vi "JoinGame.vi"(8 "error in (no error)":errorcluster, 10 "PlayerName":string, 11 "CS++GoBangServer in":refnum<class "CS++GoBangServer.lvclass">) -> (0 "error out":errorcluster, 3 "CS++GoBangServer out":refnum<class "CS++GoBangServer.lvclass">)   [LabVIEW 2014, in "GoBang.lvlib" / "CS++GoBangServer.lvclass"]
uses:
  CS++GoBangServer.lvclass
  typdefs/GameState.ctl
  CS++GoBangServer.lvclass/CS++GoBangServer.ctl
  GoBang.lvlib
panel:
  in  "Color(True=White)":bool
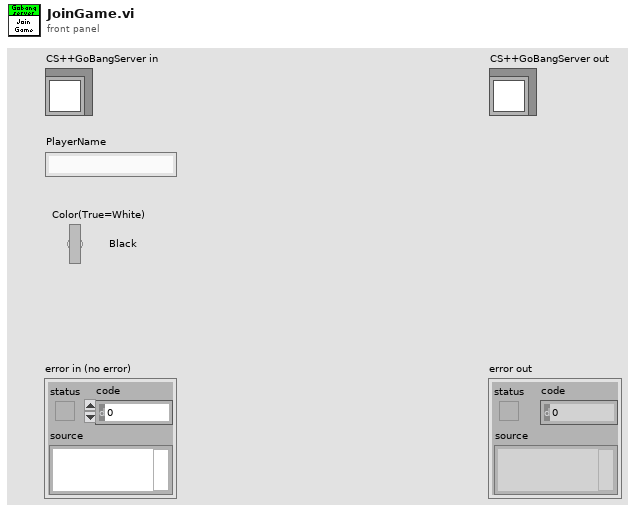
[diagram p1: front panel]
types:
  T1 = typedef "GoBang.lvlib/GameState.ctl" = enum16{"Waiting for opponent", "White to move", "Black to move", "Game over, white won", "Game over, black won"}
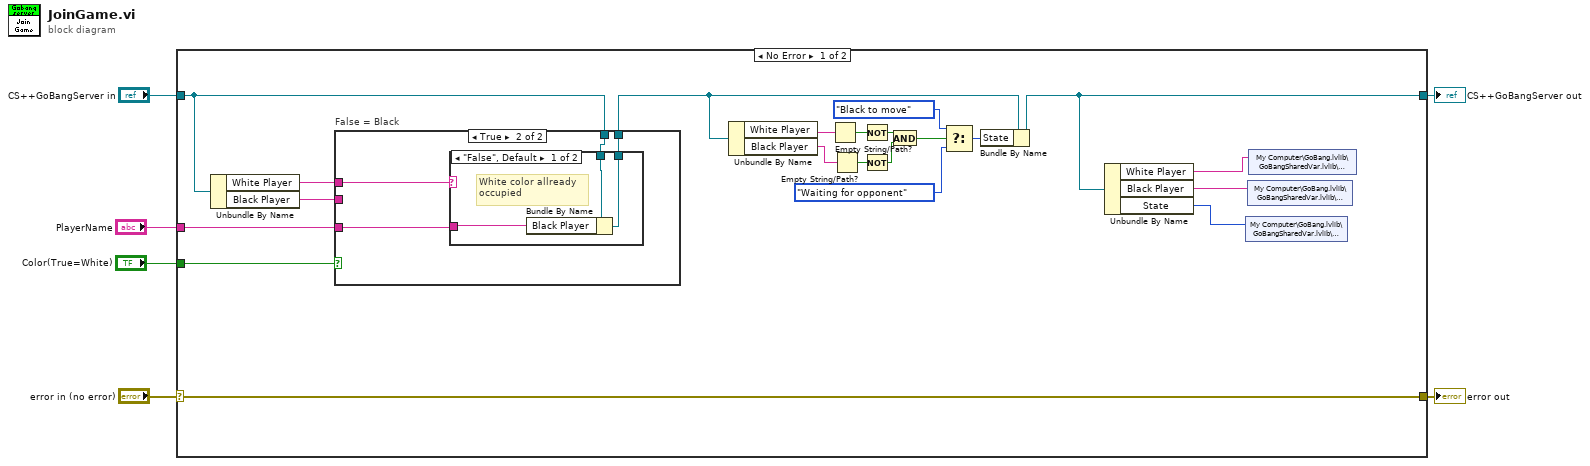
[diagram p0: block diagram]
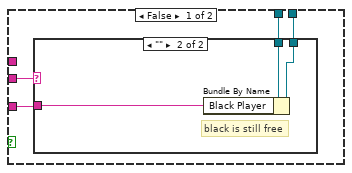
[diagram p2: hidden frame]
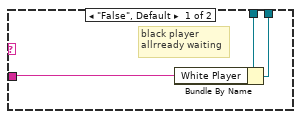
[diagram p3: hidden frame]
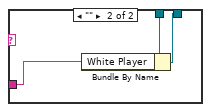
[diagram p4: hidden frame]
diagram:
  n1 = case shown="No Error" "error in (no error)" {
    selector: "error in (no error)" -> [w22 w49]
    tunnel: [w22 w49] -> w5
    tunnel: [w11 w48] -> w3
    tunnel: "CS++GoBangServer in" -> [w25 w48]
    tunnel: "Color(True=White)" -> [w27 _]
    tunnel: "PlayerName" -> [w24 _]
    frame No Error {
      n2 = Unbundle By Name(w25) -> ("White Player"=w23:string, "Black Player"=w26:string)
      n3 = case "False = Black" shown="True" w27 {
        tunnel: w26 -> [w29 _]
        tunnel: w25 -> [w31 w41]
        tunnel: [w30 w40] -> w21
        tunnel: w24 -> [w28 w39]
        tunnel: w23 -> [_ w38]
        frame False {
          n4 = case shown="\"\"" w29 {
            tunnel: w31 -> [w33 w37]
            tunnel: [w34 w36] -> w30
            tunnel: w28 -> [w32 w35]
            frame "False", Default {
              # "black player\nallrready waiting"
              n5 = Bundle By Name(cluster=w33, "White Player"=w32) -> (w34:refnum<class "CS++GoBangServer.lvclass">)
            }
            frame "" {
              # "black is still free"
              n6 = Bundle By Name(cluster=w37, "Black Player"=w35) -> (w36:refnum<class "CS++GoBangServer.lvclass">)
            }
          }
        }
        frame True {
          n7 = case shown="\"False\", Default" w38 {
            tunnel: w41 -> [w43 w47]
            tunnel: [w44 w46] -> w40
            tunnel: w39 -> [w42 w45]
            frame "False", Default {
              # "White color allready \noccupied"
              n8 = Bundle By Name(cluster=w43, "Black Player"=w42) -> (w44:refnum<class "CS++GoBangServer.lvclass">)
            }
            frame "" {
              n9 = Bundle By Name(cluster=w47, "White Player"=w45) -> (w46:refnum<class "CS++GoBangServer.lvclass">)
            }
          }
        }
      }
      n10 = Unbundle By Name(w21) -> ("White Player"=w20:string, "Black Player"=w19:string)
      n11 = Empty String/Path?(string/path=w20) -> (empty?=w17:bool)
      n12 = Empty String/Path?(string/path=w19) -> (empty?=w18:bool)
      n13 = Not(x=w17) -> (.not. x?=w16:bool)
      n14 = Not(x=w18) -> (.not. x?=w15:bool)
      n15 = And(x=w16, y=w15) -> (x .and. y?=w14:bool)
      n16 = Select(t=GameState."Black to move" ("State"), s=w14, f=GameState."Waiting for opponent" ("State")) -> (s? t:f=w10:T1)
      n17 = Bundle By Name(cluster=w21, "State"=w10) -> (w11:refnum<class "CS++GoBangServer.lvclass">)
      n18 = Unbundle By Name(w11) -> ("White Player"=w8:string, "Black Player"=w9:string, "State"=w7:T1)
      n19 = shared-variable "My Computer\\GoBang.lvlib\\GoBangSharedVar.lvlib\\GameState"(w7) -> ()  [unwired: 1 in, 1 out]
      n20 = shared-variable "My Computer\\GoBang.lvlib\\GoBangSharedVar.lvlib\\BlackPlayer"(w9) -> ()  [unwired: 1 in, 1 out]
      n21 = shared-variable "My Computer\\GoBang.lvlib\\GoBangSharedVar.lvlib\\WhitePlayer"(w8) -> ()  [unwired: 1 in, 1 out]
    }
    frame Error {
    }
  }
  "error out" <- w5
  "CS++GoBangServer out" <- w3
